vi "Constants.vi"() -> ()   [LabVIEW 2019, in "Resource Manager.lvlib"]
uses:
  Resource Manager.lvlib
panel:
  in  "module path":path
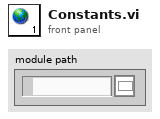
[diagram p1: front panel]
diagram:
